vi "DO DynData File Reading.vi"(8 "error in":errorcluster, 11 "Data":T1[](array[typedef])) -> (0 "error out":errorcluster, 3 "Data":T1[](array[typedef]))   [LabVIEW 2024]
doc: "All Rights Reserved © 2017 SyncSols"
uses:
  Digital Dynamic Cluster.ctl
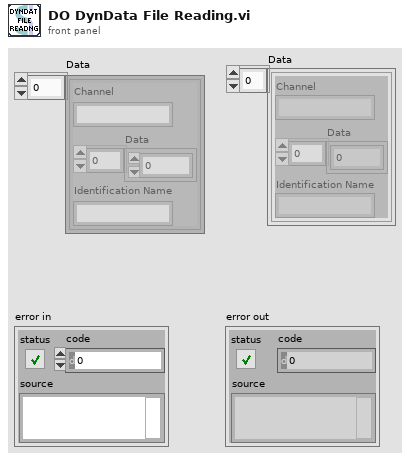
[diagram p1: front panel]
types:
  T1 = typedef "Digital Dynamic Cluster.ctl" = cluster{"Channel":string, "Data":u8[], "Identification Name":string}
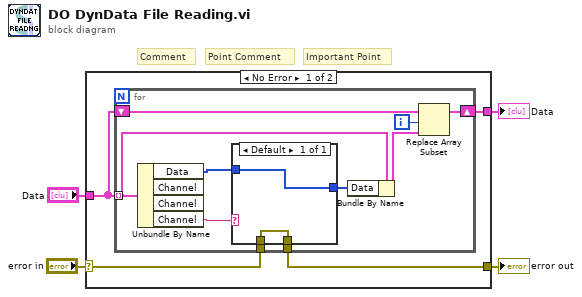
[diagram p0: block diagram]
diagram:
  # "Important Point"
  # "Point Comment"
  # "Comment"
  n1 = case shown="No Error" "error in" {
    selector: "error in" -> [w8 w22]
    tunnel: [w7 w22] -> w4
    tunnel: [w6 w21] -> w2
    tunnel: "Data" -> [w5 w21]
    frame No Error {
      n2 = for {
        tunnel: w5 -> [w11] mode=indexing
        tunnel: w8 -> [w17]
        tunnel: [w16] -> w7
        shift-right: [w12] -> w6
        shift-left: w5 -> [w14]
        i -> [w13]
        n3 = Unbundle By Name(w11) -> ("Data"=w15:u8[], "Channel"=w18:string)  [unwired: 2 out]
        n4 = case shown="Default" w18 {
          tunnel: w17 -> [w20]
          tunnel: [w20] -> w16
          tunnel: [w19] -> w10
          tunnel: w15 -> [w19]
          frame Default {
          }
        }
        n5 = Bundle By Name(cluster=w11, "Data"=w10) -> (w9:T1)
        n6 = Replace Array Subset(array=w14, new element=w9, index=w13) -> (w12:T1[])
      }
    }
    frame Error {
    }
  }
  "error out" <- w4
  "Data" <- w2
